vi "SetSettings.vi"(8 "error in (no error)":errorcluster, 11 "MagSpec_Bella in":refnum<class "MagSpec_Bella.lvclass">) -> (0 "error out":errorcluster, 3 "MagSpec_Bella out":refnum<class "MagSpec_Bella.lvclass">)   [LabVIEW 2020, in "MagSpec_Bella.lvclass"]
uses:
  MagSpec_Bella.lvclass
  MagSpec_Bella.lvclass/MagSpec_Bella.ctl
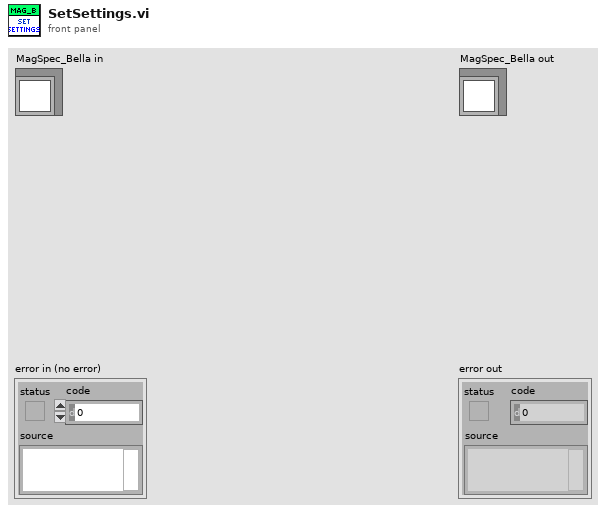
[diagram p1: front panel]
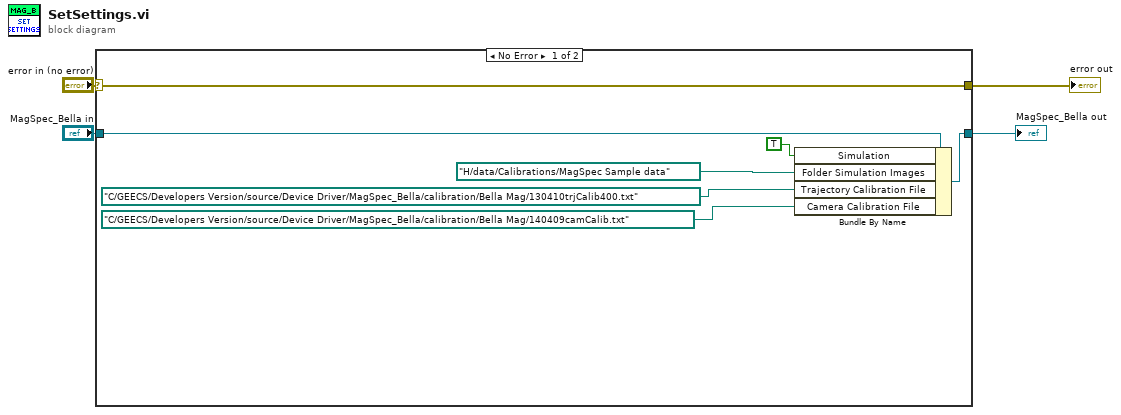
[diagram p0: block diagram]
diagram:
  n1 = case shown="No Error" "error in (no error)" {
    selector: "error in (no error)" -> [w11 w13]
    tunnel: [w11 w13] -> w3
    tunnel: [w9 w12] -> w1
    tunnel: "MagSpec_Bella in" -> [w10 w12]
    frame No Error {
      n2 = Bundle By Name(cluster=w10, "Simulation"=TRUE ("Settings.Simulation"), "Folder Simulation Images"=path "H:/data/Calibrations/MagSpec Sample data" ("Settings.Folder Simulation Images"), "Trajectory Calibration File"=path "C:/GEECS/Developers Version/source/Device Driver/MagSpec_Bella/calibration/Bella Mag/130410trjCalib400.txt" ("Settings.Calibration Files.Trajectory Calibration File"), "Camera Calibration File"=path "C:/GEECS/Developers Version/source/Device Driver/MagSpec_Bella/calibration/Bella Mag/140409camCalib.txt" ("Settings.Calibration Files.Camera Calibration File")) -> (w9:refnum<class "MagSpec_Bella.lvclass">)
    }
    frame Error {
    }
  }
  "error out" <- w3
  "MagSpec_Bella out" <- w1
